vi "Read Last Config Line 2018.vi"(6 "error in (no error)":errorcluster, 7 "Start Col":i32, 9 "Test Config path":path) -> (0 "error out":errorcluster, 1 "1d Out":string[](array[string]), 3 "2d Output":string[][](array[string]), 4 "size(s)":i32[](array[numeric]))   [LabVIEW 2020]
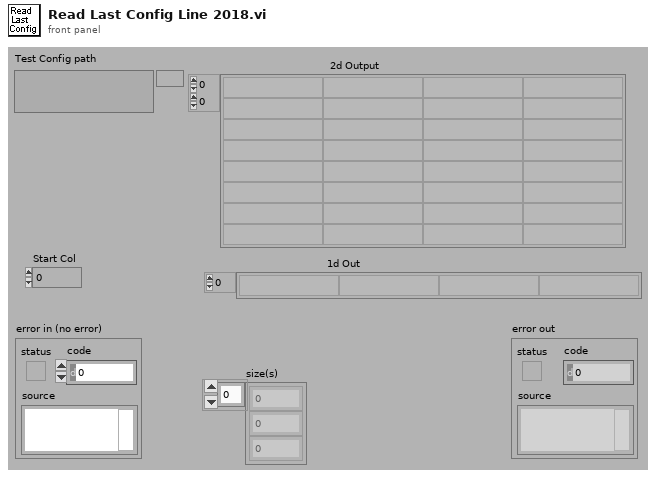
[diagram p1: front panel]
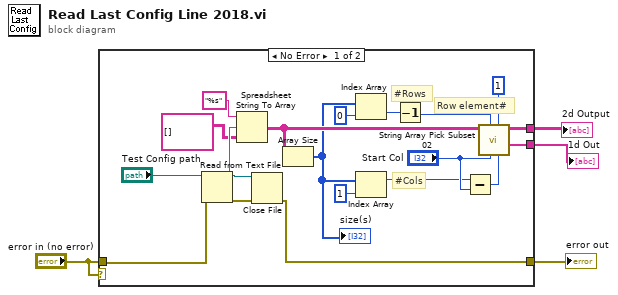
[diagram p0: block diagram]
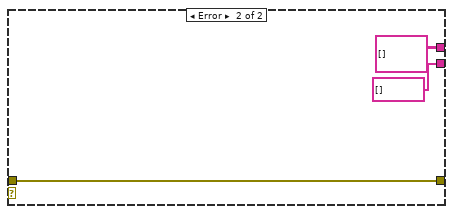
[diagram p2: hidden frame]
diagram:
  n1 = case shown="No Error" "error in (no error)" {
    tunnel: [w22 string[][] [] ("2d Output")] -> w4
    tunnel: [w14 string[] [] ("1d Out")] -> w3
    tunnel: "error in (no error)" -> [w8 w27]
    tunnel: [w5 w27] -> w2
    frame No Error {
      # "Row element#"
      # "#Cols"
      # "#Rows"
      n2 = Read from Text File(file (use dialog)="Test Config path", error in=w8) -> (refnum out=w6:refnum<file>, text=w24:string, error out=w7:errorcluster)  [unwired: 2 in, 1 out]
      n3 = Spreadsheet String To Array(format string="%s", spreadsheet string=w24, array type (2D Dbl)=string[][] [] ("Array")) -> (array=w20:string[][])  [unwired: 1 out]
      n4 = Close File(refnum=w6, error in=w7) -> (error out=w5:errorcluster)  [unwired: 1 out]
      n5 = Array Size(array=w20) -> (size(s)=w19:i32[])
      "size(s)" <- w19
      n6 = Index Array(array=w19, index=0) -> (element=w16:i32)
      n7 = Index Array(array=w19, index=1) -> (element=w10:i32)
      n8 = Decrement(x=w16) -> (x-1=w15:i32)
      n9 = Subtract(x=w10, y="Start Col") -> (x-y=w9:i32)
      n10 = call "String Array Pick Subset 02.vi"("# of Columns"=w9, "# of Rows"=1, "Start Col"="Start Col", "Start Row"=w15, "String Array"=w20) -> ("1d Out"=w14:string[], "2d Output"=w22:string[][])  [unwired: 1 in, 4 out]
    }
    frame Error {
    }
  }
  "2d Output" <- w4
  "1d Out" <- w3
  "error out" <- w2
